vi "Read from Connection.vi"(8 "error in (no error)":errorcluster, 10 "Connection":refnum<class "IConnection.lvclass">, 11 "LogEventMessageProtocol in":refnum<class "LogEventMessageProtocol.lvclass">) -> (0 "error out":errorcluster, 2 "Data Read":string, 3 "LogEventMessageProtocol out":refnum<class "LogEventMessageProtocol.lvclass">)   [LabVIEW 2017, in "Network Sink.lvlib" / "LogEventMessageProtocol.lvclass"]
uses:
  <vilib>/gpm_packages/@cs/event-logger/Source/Network Sink/LogEventMessageProtocol/LogEventMessageProtocol.lvclass
  <vilib>/gpm_packages/@cs/Network-sink/Source/Network Interface/IConnection/IConnection.lvclass
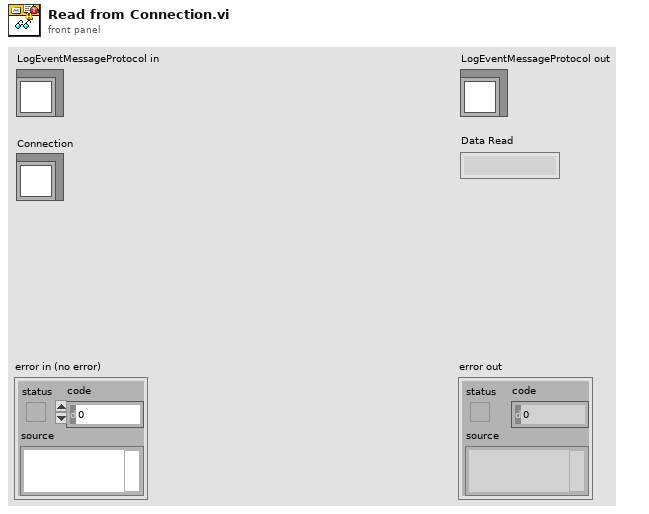
[diagram p1: front panel]
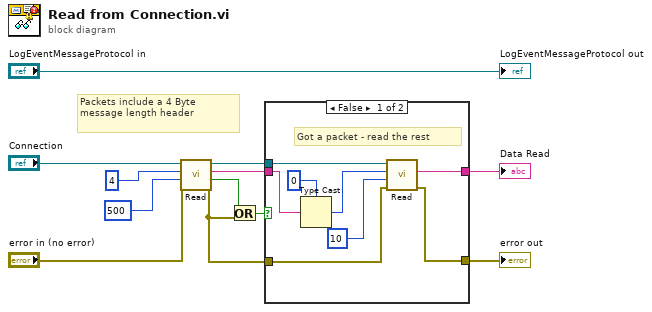
[diagram p0: block diagram]
diagram:
  # "Packets include a 4 Byte message length header"
  n1 = call-dynamic "Read.vi"("error in (no error)"="error in (no error)", "Timeout (ms)"=500, "Bytes to Read"=4, "IConnection in"="Connection") -> ("error out"=w6:errorcluster, "TimeOut?"=w5:bool, "Data"=w4:string, "IConnection out"=w3:refnum<class "IConnection.lvclass">)  [unwired: 4 in]
  n2 = Or(x=w5, y=w6) -> (x .or. y?=w7:bool)
  n3 = case shown="False" w7 {
    tunnel: w6 -> [w16 w21]
    tunnel: w4 -> [w19 _]
    tunnel: w3 -> [w20 _]
    tunnel: [w14 w21] -> w2
    tunnel: [w13 _] -> w1
    frame False {
      # "Got a packet - read the rest"
      n4 = Type Cast(type=0 ("Bytes to Read"), x=w19) -> (*(type *) &x=w17:i32)
      n5 = call-dynamic "Read.vi"("error in (no error)"=w16, "Timeout (ms)"=10, "Bytes to Read"=w17, "IConnection in"=w20) -> ("error out"=w14:errorcluster, "Data"=w13:string)  [unwired: 4 in, 2 out]
    }
    frame True {
    }
  }
  "error out" <- w2
  "Data Read" <- w1
  "LogEventMessageProtocol out" <- "LogEventMessageProtocol in"
